vi "DAQ Konfig.vi"(6 "Virtual Dev Error (F)":bool, 7 "Set up":T1, 8 "error in":errorcluster, 10 "Real physical channels":tag) -> (0 "error out":errorcluster, 3 "Refs Data out":T2)   [LabVIEW 2013]
doc: "Konfiguruje obsługę karty\nwirtualnej lub rzeczywistej\ndo wykonania pomiaru pojedynczej wartości typu double"
uses:
  inne pliki/RefData.ctl
  inne pliki/DevSetUp.ctl
  <vilib>/DAQmx/create/channels.llb/DAQmx Create Channel (AI-Voltage-Basic).vi
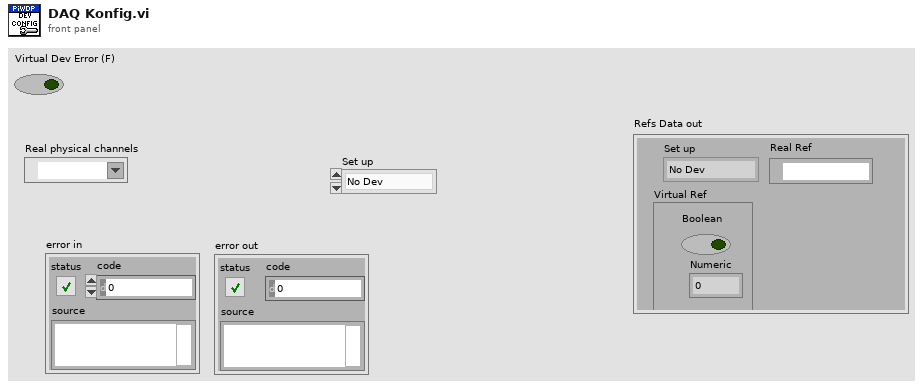
[diagram p1: front panel]
types:
  T1 = typedef "DevSetUp.ctl" = enum16{"No Dev", "Virtual Dev", "Real Dev"}
  T2 = typedef "RefData.ctl" = cluster{"Virtual Ref":cluster{"Numeric":dbl, "Boolean":bool}, "Real Ref":refnum<k21>, "Set up":T1}
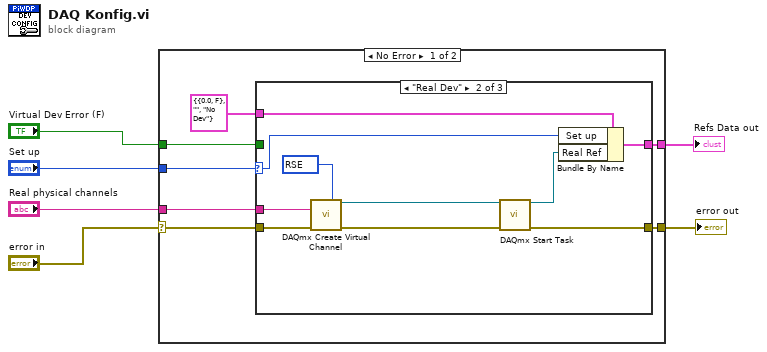
[diagram p0: block diagram]
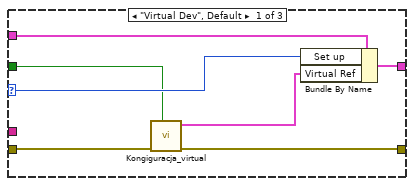
[diagram p2: hidden frame]
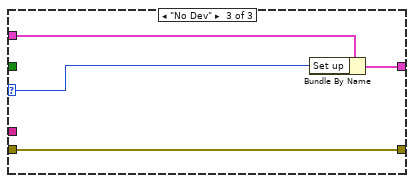
[diagram p3: hidden frame]
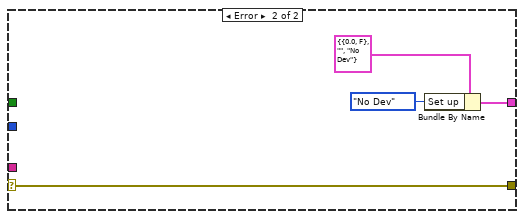
[diagram p4: hidden frame]
diagram:
  n1 = case shown="No Error" "error in" {
    selector: "error in" -> [w11 w38]
    tunnel: "Real physical channels" -> [w13 _]
    tunnel: [w12 w38] -> w5
    tunnel: "Set up" -> [w10 _]
    tunnel: [w8 w37] -> w2
    tunnel: "Virtual Dev Error (F)" -> [w7 _]
    frame No Error {
      n2 = case shown="\"Real Dev\"" w10 {
        selector: w10 -> [w15 w23 w31]
        tunnel: w13 -> [_ w29 _]
        tunnel: [w19 w26 w34] -> w12
        tunnel: w11 -> [w20 w25 w34]
        tunnel: T2 {"Virtual Ref"={"Numeric"=0.0, "Boolean"=FALSE}, "Real Ref"="", "Set up"=enum."No Dev"} ("Refs Data out 2") -> [w17 w24 w32]
        tunnel: [w18 w21 w33] -> w8
        tunnel: w7 -> [w14 _ _]
        frame "Virtual Dev", Default {
          n3 = call "Kongiguracja_virtual.vi"("Error Generate"=w14, "error in (no error)"=w20) -> ("error out"=w19:errorcluster, "Reference out"=w16:cluster{"Numeric":dbl, "Boolean":bool})  [unwired: 8 in]
          n4 = Bundle By Name(cluster=w17, "Set up"=w15, "Virtual Ref"=w16) -> (w18:T2)
        }
        frame "Real Dev" {
          w30 = 10083 items=["default"=-1, "RSE"=10083, "NRSE"=10078, "Differential"=10106, "Pseudodifferential"=12529] ("input terminal configuration")
          n5 = call-poly <vilib>:"DAQmx Create Virtual Channel.vi"("input terminal configuration"=w30, "physical channels"=w29, "error in"=w25) -> ("task out"=w28:refnum<k21>, "error out"=w27:errorcluster)  [unwired: 11 in]
          n6 = call <vilib>:"DAQmx Start Task.vi"("task/channels in"=w28, "error in"=w27) -> ("task out"=w22:refnum<k21>, "error out"=w26:errorcluster)  [unwired: 12 in]
          n7 = Bundle By Name(cluster=w24, "Set up"=w23, "Real Ref"=w22) -> (w21:T2)
        }
        frame "No Dev" {
          n8 = Bundle By Name "Bundle By Name"(cluster=w32, "Set up"=w31) -> (w33:T2)
        }
      }
    }
    frame Error {
      n9 = Bundle By Name(cluster=T2 {"Virtual Ref"={"Numeric"=0.0, "Boolean"=FALSE}, "Real Ref"="", "Set up"=enum."No Dev"} ("Refs Data out 2"), "Set up"=DevSetUp."No Dev") -> (w37:T2)
    }
  }
  "error out" <- w5
  "Refs Data out" <- w2
